vi "Find Swallow Start-End.vi"(10 "Times":string[](array[string]), 11 "Labels":string[](array[string])) -> (2 "Times":string[](array[string]), 3 "Event Names":string[](array[string]))   [LabVIEW 2020]
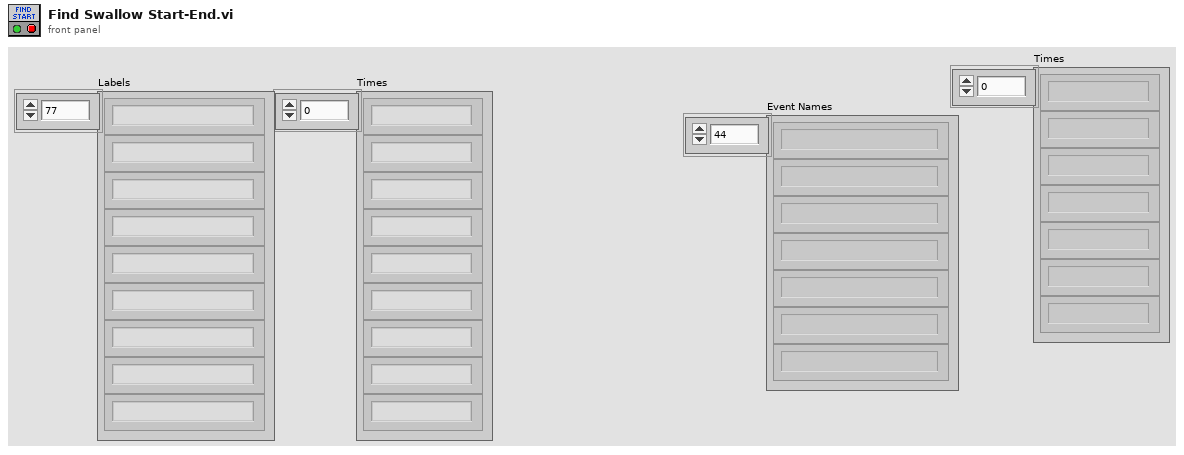
[diagram p1: front panel]
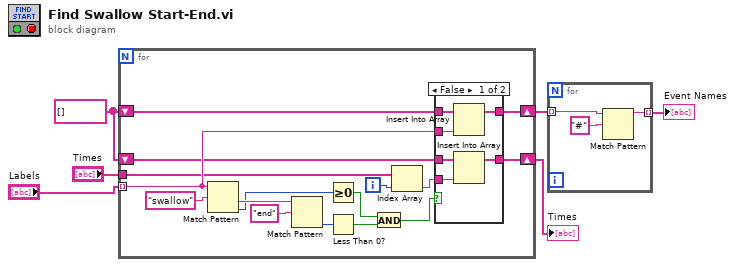
[diagram p0: block diagram]
diagram:
  w4 = string[] []
  n1 = for {
    tunnel: "Labels" -> [w13] mode=indexing
    shift-right: [w12] -> w2
    shift-left: w4 -> [w14]
    shift-right: [w9] -> w1
    shift-left: w4 -> [w10]
    tunnel: "Times" -> [w11]
    i -> [w7]
    n2 = Match Pattern(string=w13, regular expression="swallow") -> (after substring=w17:string, offset past match=w16:i32)  [unwired: 1 in, 2 out]
    n3 = Match Pattern(string=w17, regular expression="end") -> (offset past match=w20:i32)  [unwired: 1 in, 3 out]
    n4 = Greater Or Equal To 0?(x=w16) -> (x >= 0?=w15:bool)
    n5 = Less Than 0?(x=w20) -> (x < 0?=w19:bool)
    n6 = And(x=w15, y=w19) -> (x .and. y?=w18:bool)
    n7 = Index Array(array=w11, index=w7) -> (element=w8:string)
    n8 = case shown="False" w18 {
      tunnel: w14 -> [w28 w30]
      tunnel: w13 -> [w27 _]
      tunnel: [w26 w30] -> w12
      tunnel: w10 -> [w25 w29]
      tunnel: [w24 w29] -> w9
      tunnel: w8 -> [w23 _]
      frame False {
        n9 = Insert Into Array(array=w28, new element=w27) -> (w26:string[])  [unwired: 1 in]
        n10 = Insert Into Array(array=w25, new element=w23) -> (w24:string[])  [unwired: 1 in]
      }
      frame True {
      }
    }
  }
  "Times" <- w1
  n11 = for {
    tunnel: [w32] -> w6 mode=indexing
    tunnel: w2 -> [w31] mode=indexing
    n12 = Match Pattern(string=w31, regular expression="#") -> (before substring=w32:string)  [unwired: 1 in, 3 out]
  }
  "Event Names" <- w6
